vi "PowerCycleSensors.vi"(8 "error in":errorcluster) -> (0 "error out":errorcluster)   [LabVIEW 2014]
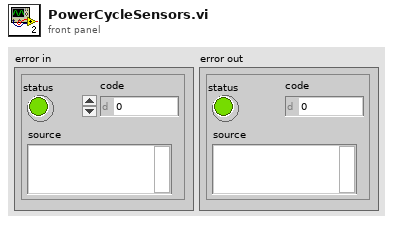
[diagram p1: front panel]
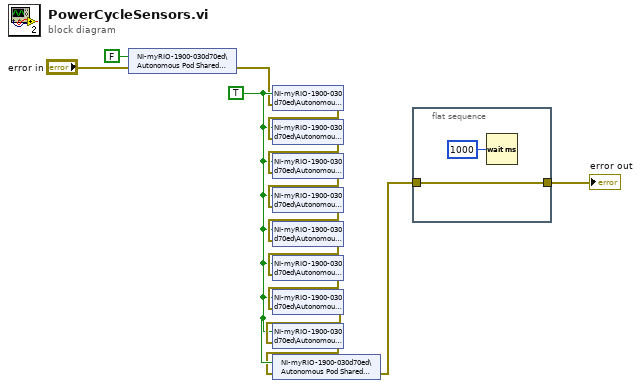
[diagram p0: block diagram]
diagram:
  w7 = TRUE
  n1 = shared-variable "NI-myRIO-1900-030d70ed\\Autonomous Pod Shared Variables.lvlib\\ResetSensor"(FALSE ("ResetSensor"), error in="error in") -> (error out=w1:errorcluster)
  n2 = shared-variable "NI-myRIO-1900-030d70ed\\Autonomous Pod Shared Variables.lvlib\\ToF1"(w7, error in=w1) -> (error out=w14:errorcluster)
  n3 = shared-variable "NI-myRIO-1900-030d70ed\\Autonomous Pod Shared Variables.lvlib\\ToF2"(w7, error in=w14) -> (error out=w13:errorcluster)
  n4 = shared-variable "NI-myRIO-1900-030d70ed\\Autonomous Pod Shared Variables.lvlib\\ToF3"(w7, error in=w13) -> (error out=w12:errorcluster)
  n5 = shared-variable "NI-myRIO-1900-030d70ed\\Autonomous Pod Shared Variables.lvlib\\ToF4"(w7, error in=w12) -> (error out=w11:errorcluster)
  n6 = shared-variable "NI-myRIO-1900-030d70ed\\Autonomous Pod Shared Variables.lvlib\\ToF5"(w7, error in=w11) -> (error out=w10:errorcluster)
  n7 = shared-variable "NI-myRIO-1900-030d70ed\\Autonomous Pod Shared Variables.lvlib\\ToF6"(w7, error in=w10) -> (error out=w9:errorcluster)
  n8 = shared-variable "NI-myRIO-1900-030d70ed\\Autonomous Pod Shared Variables.lvlib\\ToF7"(w7, error in=w9) -> (error out=w8:errorcluster)
  n9 = shared-variable "NI-myRIO-1900-030d70ed\\Autonomous Pod Shared Variables.lvlib\\ToF8"(w7, error in=w8) -> (error out=w6:errorcluster)
  n10 = shared-variable "NI-myRIO-1900-030d70ed\\Autonomous Pod Shared Variables.lvlib\\SensePower"(w7, error in=w6) -> (error out=w4:errorcluster)
  n11 = flat-sequence {
    tunnel: [w16] -> w5
    tunnel: w4 -> [w16]
    frame #0 {
      n12 = Wait (ms)(milliseconds to wait=u32 1000) -> ()  [unwired: 1 out]
    }
  }
  "error out" <- w5
